vi "FaceSymbol2Color2.vi"(9 "Pict Ring":T1, 10 "Pict Ring 2":T1, 11 "Array":string[](array[string])) -> (3 "String":string)   [LabVIEW 2017]
doc: "Take the string (char) array of 6 colors (e.g. \"wgrboy\") and identify the colors of the faces' enum: \nUF might be \"wr\"(== colors white and red).\nOr you enter string (char) array of 6 symbols (enum) (e.g. \"ULFRBD\") that is translated into a sting as \"UR\"\n\nThe inputs #2 an #3 accept the ring control items corresponding to the facelets.\n\nSee also VI \"FaceSymbol2Color3.vi\""
uses:
  FaceletColorRing.ctl
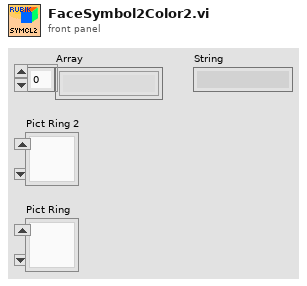
[diagram p1: front panel]
types:
  T1 = typedef "FaceletColorRing.ctl" = u16
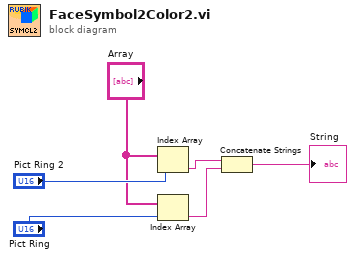
[diagram p0: block diagram]
diagram:
  n1 = Index Array(array="Array", index="Pict Ring 2") -> (element=w4:string)
  n2 = Index Array(array="Array", index="Pict Ring") -> (element=w1:string)
  n3 = Concatenate Strings(w4, w1) -> (→"String":string)
